vi "Enable UI.vi"(8 "error in (no error)":errorcluster, 11 "Function UI in":refnum<class "Controller UI.lvclass">) -> (0 "error out":errorcluster, 3 "Function UI out":refnum<class "Controller UI.lvclass">)   [LabVIEW 2016, in "Controller UI.lvlib" / "Controller UI.lvclass"]
uses:
  <userlib>/Common Components/Controller UI/Controller UI.lvclass
  <userlib>/Common Components/Controller UI/Controller UI.lvclass/Controller UI.ctl
  <userlib>/Common Components/Controller UI/Accessors/Read Load New Function.vi
  <userlib>/Common Components/Controller UI/Accessors/Read Function.vi
  <userlib>/Common Components/Controller UI/Accessors/Read Show FP_.vi
  <userlib>/Common Components/User Interface/UI.lvclass
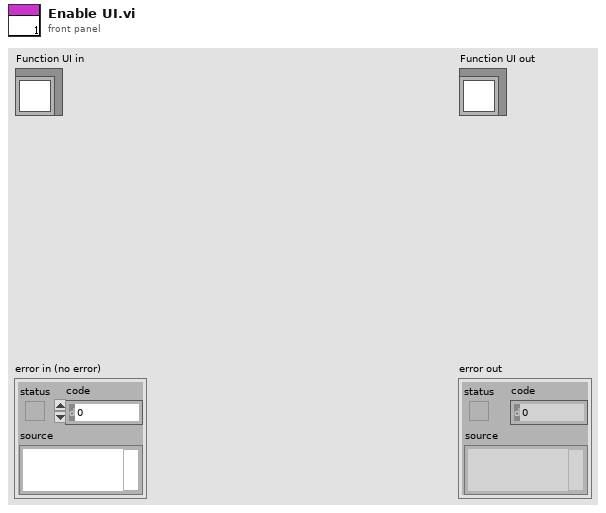
[diagram p1: front panel]
types:
  T1 = enum8{"Enabled", "Disabled", "Disabled and Grayed Out"}
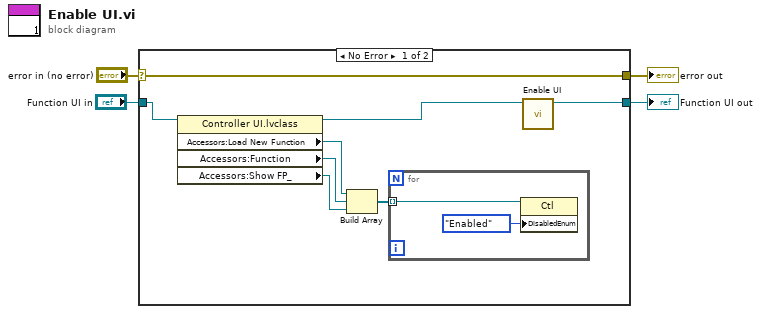
[diagram p0: block diagram]
diagram:
  n1 = case shown="No Error" "error in (no error)" {
    selector: "error in (no error)" -> [w12 w16]
    tunnel: [w12 w16] -> w3
    tunnel: [w6 w15] -> w1
    tunnel: "Function UI in" -> [w8 w15]
    frame No Error {
      n2 = property class="Controller UI.lvclass"(reference=w8) -> (reference out=w7:refnum<class "Controller UI.lvclass">, "Accessors:Load New Function"=w5:refnum<vi>, "Accessors:Function"=w9:refnum<vi>, "Accessors:Show FP_"=w10:refnum<vi>)  [unwired: 1 in, 1 out]
      n3 = Build Array(w5, w9, w10) -> (w11:refnum<vi>[])
      n4 = for {
        tunnel: w11 -> [w14] mode=indexing
        n5 = property class="Ctl"(reference=w14, "DisabledEnum"=T1."Enabled" ("Disabled")) -> ()  [unwired: 1 in, 2 out]
      }
      n6 = call-parent "Enable UI.vi"("UI in"=w7) -> ("UI out"=w6:refnum<class "Controller UI.lvclass">)  [unwired: 9 in, 1 out]
    }
    frame Error {
    }
  }
  "error out" <- w3
  "Function UI out" <- w1
